vi "FlattenData.vi"(3 "Physical Quantities":T3, 4 "All data after scaling":T4, 5 "All DAQ channels":T2) -> (1 "Flattened data":T1)   [LabVIEW 2020, in "SignalConverson.lvlib"]
uses:
  SignalConverson.lvlib
  ScaledData.ctl
  Measrured TrapXYZ.ctl
  Data Before Angle Compensation.ctl
  Angle compensated data.ctl
  XYZ Signals.ctl
  Set TrapXYZ.ctl
  Initialization/Physical Quantitites.ctl
  DAQChannelRawData.ctl
  FlattenedData.ctl
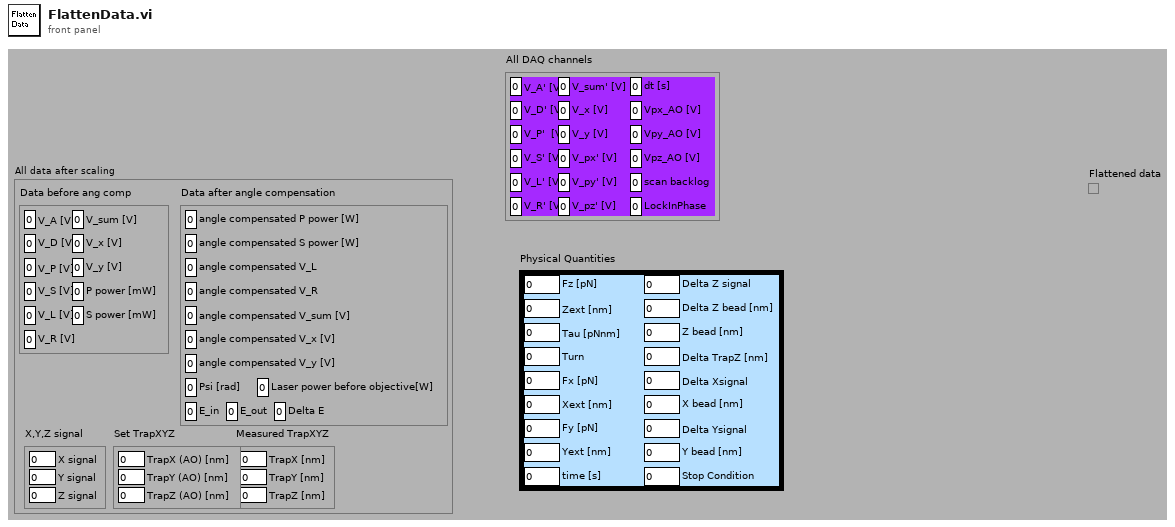
[diagram p1: front panel]
types:
  T1 = typedef "SignalConverson.lvlib/FlattenedData.ctl" = cluster{"V_A' [V]":dbl, "V_D' [V]":dbl, "V_P'  [V]":dbl, "V_S' [V]":dbl, "V_L' [V]":dbl, "V_R' [V]":dbl, "V_sum' [V]":dbl, "V_x [V]":dbl, "V_y [V]":dbl, "V_px' [V]":dbl, "V_py' [V]":dbl, "V_pz' [V]":dbl, "dt [s]":dbl, "Vpx_AO [V]":dbl, "Vpy_AO [V]":dbl, "Vpz_AO [V]":dbl, "scan backlog":dbl, "LockInPhase":dbl, "TrapX [nm]":dbl, "TrapY [nm]":dbl, "TrapZ [nm]":dbl, "V_A [V]":dbl, "V_D [V]":dbl, "V_P [V]":dbl, "V_S [V]":dbl, "V_L [V]":dbl, "V_R [V]":dbl, "V_sum [V]":dbl, "V_x [V]":dbl, "V_y [V]":dbl, "P power [mW]":dbl, "S power [mW]":dbl, "angle compensated P power [W]":dbl, "angle compensated S power [W]":dbl, "angle compensated V_L":dbl, "angle compensated V_R":dbl, "angle compensated V_sum [V]":dbl, "angle compensated V_x [V]":dbl, "angle compensated V_y [V]":dbl, "Psi [rad]":dbl, "Laser power before objective[W]":dbl, "E_in":dbl, "E_out":dbl, "Delta E":dbl, "X signal":dbl, "Y signal":dbl, "Z signal":dbl, "TrapX (AO) [nm]":dbl, "TrapY (AO) [nm]":dbl, "TrapZ (AO) [nm]":dbl, "Fz [pN]":dbl, "Zext [nm]":dbl, "Tau [pNnm]":dbl, "Turn":dbl, "Fx [pN]":dbl, "Xext [nm]":dbl, "Fy [pN]":dbl, "Yext [nm]":dbl, "time [s]":dbl, "Delta Z signal":dbl, "Delta Z bead [nm]":dbl, "Z bead [nm]":dbl, "Delta TrapZ [nm]":dbl, "Delta Xsignal":dbl, "X bead [nm]":dbl, "Delta Ysignal":dbl, "Y bead [nm]":dbl, "Stop Condition":dbl}
  T2 = typedef "SignalConverson.lvlib/DAQChannelRawData.ctl" = cluster{"V_A' [V]":dbl, "V_D' [V]":dbl, "V_P'  [V]":dbl, "V_S' [V]":dbl, "V_L' [V]":dbl, "V_R' [V]":dbl, "V_sum' [V]":dbl, "V_x [V]":dbl, "V_y [V]":dbl, "V_px' [V]":dbl, "V_py' [V]":dbl, "V_pz' [V]":dbl, "dt [s]":dbl, "Vpx_AO [V]":dbl, "Vpy_AO [V]":dbl, "Vpz_AO [V]":dbl, "scan backlog":u32, "LockInPhase":dbl}
  T3 = typedef "SignalConverson.lvlib/Physical Quantitites.ctl" = cluster{"Fz [pN]":dbl, "Zext [nm]":dbl, "Tau [pNnm]":dbl, "Turn":dbl, "Fx [pN]":dbl, "Xext [nm]":dbl, "Fy [pN]":dbl, "Yext [nm]":dbl, "time [s]":dbl, "Delta Z signal":dbl, "Delta Z bead [nm]":dbl, "Z bead [nm]":dbl, "Delta TrapZ [nm]":dbl, "Delta Xsignal":dbl, "X bead [nm]":dbl, "Delta Ysignal":dbl, "Y bead [nm]":dbl, "Stop Condition":dbl}
  T4 = typedef "SignalConverson.lvlib/ScaledData.ctl" = cluster{"Measured TrapXYZ":T5, "Data before ang comp":T6, "Data after angle compensation":T7, "X,Y,Z signal":T8, "Set TrapXYZ":T9}
  T5 = typedef "SignalConverson.lvlib/Measrured TrapXYZ.ctl" = cluster{"TrapX [nm]":dbl, "TrapY [nm]":dbl, "TrapZ [nm]":dbl}
  T6 = typedef "SignalConverson.lvlib/Data Before Angle Compensation.ctl" = cluster{"V_A [V]":dbl, "V_D [V]":dbl, "V_P [V]":dbl, "V_S [V]":dbl, "V_L [V]":dbl, "V_R [V]":dbl, "V_sum [V]":dbl, "V_x [V]":dbl, "V_y [V]":dbl, "P power [mW]":dbl, "S power [mW]":dbl}
  T7 = typedef "SignalConverson.lvlib/Angle compensated data.ctl" = cluster{"angle compensated P power [W]":dbl, "angle compensated S power [W]":dbl, "angle compensated V_L":dbl, "angle compensated V_R":dbl, "angle compensated V_sum [V]":dbl, "angle compensated V_x [V]":dbl, "angle compensated V_y [V]":dbl, "Psi [rad]":dbl, "Laser power before objective[W]":dbl, "E_in":dbl, "E_out":dbl, "Delta E":dbl}
  T8 = typedef "SignalConverson.lvlib/XYZ Signals.ctl" = cluster{"X signal":dbl, "Y signal":dbl, "Z signal":dbl}
  T9 = typedef "SignalConverson.lvlib/Set TrapXYZ.ctl" = cluster{"TrapX (AO) [nm]":dbl, "TrapY (AO) [nm]":dbl, "TrapZ (AO) [nm]":dbl}
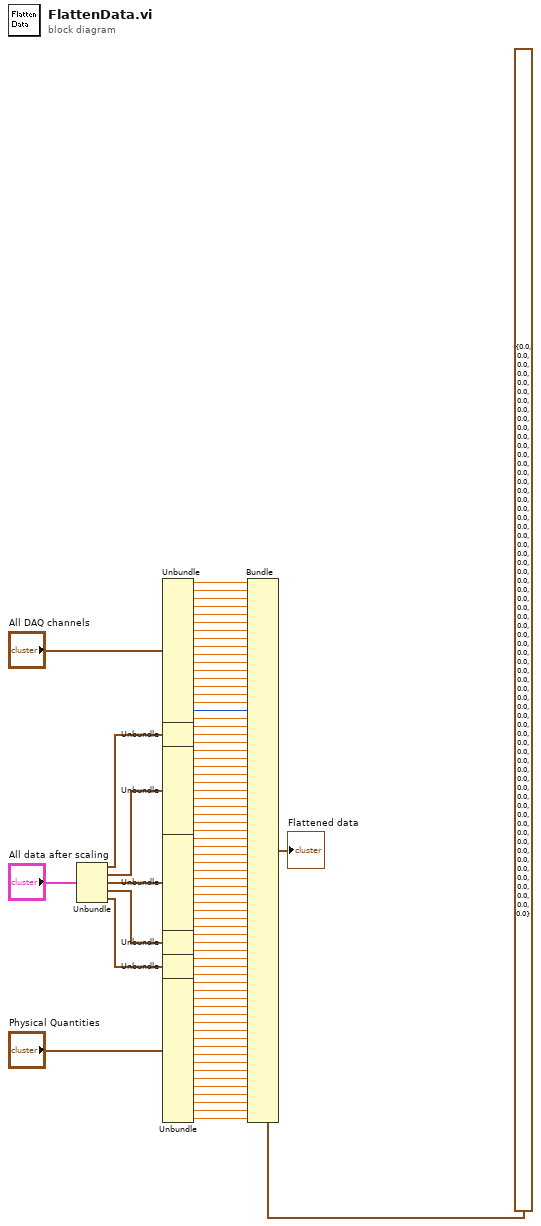
[diagram p0: block diagram]
diagram:
  n1 = Unbundle("All data after scaling") -> ("Measured TrapXYZ"=w60:T5, "Data before ang comp"=w56:T6, "Data after angle compensation"=w44:T7, "X,Y,Z signal"=w31:T8, "Set TrapXYZ"=w27:T9)
  n2 = Unbundle("All DAQ channels") -> ("V_A' [V]"=w77:dbl, "V_D' [V]"=w76:dbl, "V_P'  [V]"=w75:dbl, "V_S' [V]"=w74:dbl, "V_L' [V]"=w73:dbl, "V_R' [V]"=w72:dbl, "V_sum' [V]"=w71:dbl, "V_x [V]"=w70:dbl, "V_y [V]"=w69:dbl, "V_px' [V]"=w68:dbl, "V_py' [V]"=w67:dbl, "V_pz' [V]"=w66:dbl, "dt [s]"=w65:dbl, "Vpx_AO [V]"=w64:dbl, "Vpy_AO [V]"=w63:dbl, "Vpz_AO [V]"=w62:dbl, "scan backlog"=w3:u32, "LockInPhase"=w2:dbl)
  n3 = Unbundle(w60) -> ("TrapX [nm]"=w59:dbl, "TrapY [nm]"=w58:dbl, "TrapZ [nm]"=w57:dbl)
  n4 = Unbundle(w56) -> ("V_A [V]"=w55:dbl, "V_D [V]"=w54:dbl, "V_P [V]"=w53:dbl, "V_S [V]"=w52:dbl, "V_L [V]"=w51:dbl, "V_R [V]"=w50:dbl, "V_sum [V]"=w49:dbl, "V_x [V]"=w48:dbl, "V_y [V]"=w47:dbl, "P power [mW]"=w46:dbl, "S power [mW]"=w45:dbl)
  n5 = Unbundle(w44) -> ("angle compensated P power [W]"=w43:dbl, "angle compensated S power [W]"=w42:dbl, "angle compensated V_L"=w41:dbl, "angle compensated V_R"=w40:dbl, "angle compensated V_sum [V]"=w39:dbl, "angle compensated V_x [V]"=w38:dbl, "angle compensated V_y [V]"=w37:dbl, "Psi [rad]"=w36:dbl, "Laser power before objective[W]"=w35:dbl, "E_in"=w34:dbl, "E_out"=w33:dbl, "Delta E"=w32:dbl)
  n6 = Unbundle(w31) -> ("X signal"=w30:dbl, "Y signal"=w29:dbl, "Z signal"=w28:dbl)
  n7 = Unbundle(w27) -> ("TrapX (AO) [nm]"=w26:dbl, "TrapY (AO) [nm]"=w25:dbl, "TrapZ (AO) [nm]"=w24:dbl)
  n8 = Unbundle("Physical Quantities") -> ("Fz [pN]"=w5:dbl, "Zext [nm]"=w6:dbl, "Tau [pNnm]"=w7:dbl, "Turn"=w8:dbl, "Fx [pN]"=w9:dbl, "Xext [nm]"=w10:dbl, "Fy [pN]"=w11:dbl, "Yext [nm]"=w12:dbl, "time [s]"=w13:dbl, "Delta Z signal"=w14:dbl, "Delta Z bead [nm]"=w15:dbl, "Z bead [nm]"=w16:dbl, "Delta TrapZ [nm]"=w17:dbl, "Delta Xsignal"=w18:dbl, "X bead [nm]"=w19:dbl, "Delta Ysignal"=w20:dbl, "Y bead [nm]"=w21:dbl, "Stop Condition"=w22:dbl)
  n9 = Bundle(cluster=T1 {"V_A' [V]"=0.0, "V_D' [V]"=0.0, "V_P'  [V]"=0.0, "V_S' [V]"=0.0, "V_L' [V]"=0.0, "V_R' [V]"=0.0, "V_sum' [V]"=0.0, "V_x [V]"=0.0, "V_y [V]"=0.0, "V_px' [V]"=0.0, "V_py' [V]"=0.0, "V_pz' [V]"=0.0, "dt [s]"=0.0, "Vpx_AO [V]"=0.0, "Vpy_AO [V]"=0.0, "Vpz_AO [V]"=0.0, "scan backlog"=0.0, "LockInPhase"=0.0, "TrapX [nm]"=0.0, "TrapY [nm]"=0.0, "TrapZ [nm]"=0.0, "V_A [V]"=0.0, "V_D [V]"=0.0, "V_P [V]"=0.0, "V_S [V]"=0.0, "V_L [V]"=0.0, "V_R [V]"=0.0, "V_sum [V]"=0.0, "V_x [V]"=0.0, "V_y [V]"=0.0, "P power [mW]"=0.0, "S power [mW]"=0.0, "angle compensated P power [W]"=0.0, "angle compensated S power [W]"=0.0, "angle compensated V_L"=0.0, "angle compensated V_R"=0.0, "angle compensated V_sum [V]"=0.0, "angle compensated V_x [V]"=0.0, "angle compensated V_y [V]"=0.0, "Psi [rad]"=0.0, "Laser power before objective[W]"=0.0, "E_in"=0.0, "E_out"=0.0, "Delta E"=0.0, "X signal"=0.0, "Y signal"=0.0, "Z signal"=0.0, "TrapX (AO) [nm]"=0.0, "TrapY (AO) [nm]"=0.0, "TrapZ (AO) [nm]"=0.0, "Fz [pN]"=0.0, "Zext [nm]"=0.0, "Tau [pNnm]"=0.0, "Turn"=0.0, "Fx [pN]"=0.0, "Xext [nm]"=0.0, "Fy [pN]"=0.0, "Yext [nm]"=0.0, "time [s]"=0.0, "Delta Z signal"=0.0, "Delta Z bead [nm]"=0.0, "Z bead [nm]"=0.0, "Delta TrapZ [nm]"=0.0, "Delta Xsignal"=0.0, "X bead [nm]"=0.0, "Delta Ysignal"=0.0, "Y bead [nm]"=0.0, "Stop Condition"=0.0} ("Flattened data 2"), "V_A' [V]"=w77, "V_D' [V]"=w76, "V_P'  [V]"=w75, "V_S' [V]"=w74, "V_L' [V]"=w73, "V_R' [V]"=w72, "V_sum' [V]"=w71, "V_x [V]"=w70, "V_y [V]"=w69, "V_px' [V]"=w68, "V_py' [V]"=w67, "V_pz' [V]"=w66, "dt [s]"=w65, "Vpx_AO [V]"=w64, "Vpy_AO [V]"=w63, "Vpz_AO [V]"=w62, "scan backlog"=w3, "LockInPhase"=w2, "TrapX [nm]"=w59, "TrapY [nm]"=w58, "TrapZ [nm]"=w57, "V_A [V]"=w55, "V_D [V]"=w54, "V_P [V]"=w53, "V_S [V]"=w52, "V_L [V]"=w51, "V_R [V]"=w50, "V_sum [V]"=w49, "V_x [V]"=w48, "V_y [V]"=w47, "P power [mW]"=w46, "S power [mW]"=w45, "angle compensated P power [W]"=w43, "angle compensated S power [W]"=w42, "angle compensated V_L"=w41, "angle compensated V_R"=w40, "angle compensated V_sum [V]"=w39, "angle compensated V_x [V]"=w38, "angle compensated V_y [V]"=w37, "Psi [rad]"=w36, "Laser power before objective[W]"=w35, "E_in"=w34, "E_out"=w33, "Delta E"=w32, "X signal"=w30, "Y signal"=w29, "Z signal"=w28, "TrapX (AO) [nm]"=w26, "TrapY (AO) [nm]"=w25, "TrapZ (AO) [nm]"=w24, "Fz [pN]"=w5, "Zext [nm]"=w6, "Tau [pNnm]"=w7, "Turn"=w8, "Fx [pN]"=w9, "Xext [nm]"=w10, "Fy [pN]"=w11, "Yext [nm]"=w12, "time [s]"=w13, "Delta Z signal"=w14, "Delta Z bead [nm]"=w15, "Z bead [nm]"=w16, "Delta TrapZ [nm]"=w17, "Delta Xsignal"=w18, "X bead [nm]"=w19, "Delta Ysignal"=w20, "Y bead [nm]"=w21, "Stop Condition"=w22) -> (→"Flattened data":T1)
